vi "get_speed_params.vi"(8 "error in (no error)":errorcluster, 11 "TrajectoryDL090201FrameScan in":refnum<class "TrajectoryDL090201FrameScan.lvclass">) -> (0 "error out":errorcluster, 1 "line-scan time":dbl[unit]=-1.0, 2 "frame rate":dbl[unit]=-1.0, 3 "TrajectoryDL090201FrameScan out":refnum<class "TrajectoryDL090201FrameScan.lvclass">, 4 "pixel-dwell time":dbl[unit]=-1e-06)   [LabVIEW 2010, in "TrajectoryDL090201FrameScan.lvclass"]
uses:
  TrajectoryDL090201FrameScan.lvclass
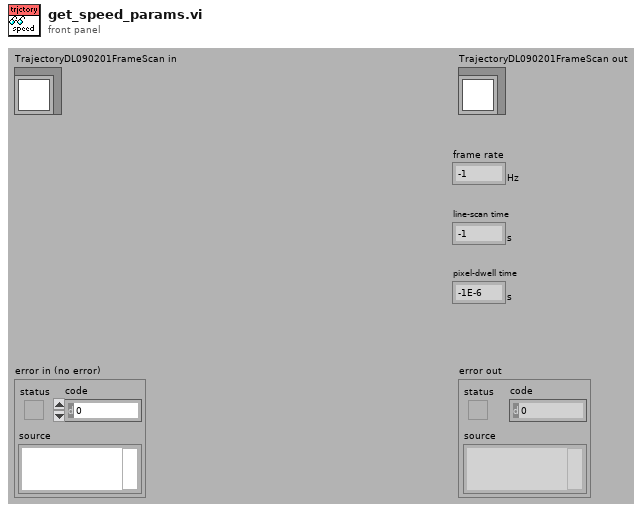
[diagram p1: front panel]
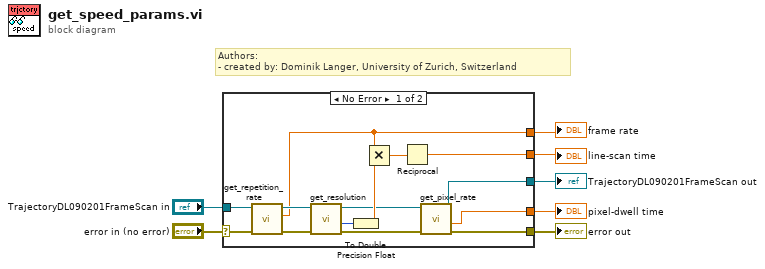
[diagram p0: block diagram]
diagram:
  # "Authors: \n- created by: Dominik Langer, University of Zurich, Switzerland"
  n1 = case shown="No Error" "error in (no error)" {
    selector: "error in (no error)" -> [w21 w23]
    tunnel: [w11 w23] -> w6
    tunnel: [w8 w22] -> w4
    tunnel: "TrajectoryDL090201FrameScan in" -> [w20 w22]
    tunnel: [w15 _] -> w3
    tunnel: [w13 _] -> w2
    tunnel: [w9 _] -> w1
    frame No Error {
      n2 = call-dynamic "get_repetition_rate.vi"("error in (no error)"=w21, "GenericTrajectory in"=w20) -> ("error out"=w18:errorcluster, "repetition rate"=w15:dbl[unit], "GenericTrajectory out"=w19:refnum<class "TrajectoryDL090201FrameScan.lvclass">)  [unwired: 7 in]
      n3 = call-dynamic "get_resolution.vi"("error in (no error)"=w18, "TrajectoryDL090201FrameScan in"=w19) -> ("error out"=w12:errorcluster, "y"=w17:i32, "TrajectoryDL090201FrameScan out"=w10:refnum<class "TrajectoryDL090201FrameScan.lvclass">)  [unwired: 6 in, 1 out]
      n4 = To Double Precision Float(number=w17) -> (double precision float=w16:dbl)
      n5 = Multiply(x=w15, y=w16) -> (x*y=w14:dbl[unit])
      n6 = Reciprocal(x=w14) -> (1/x=w13:dbl[unit])
      n7 = call-dynamic "get_pixel_rate.vi"("error in (no error)"=w12, "GenericTrajectory in"=w10) -> ("error out"=w11:errorcluster, "pixel dwell time"=w9:dbl[unit], "GenericTrajectory out"=w8:refnum<class "TrajectoryDL090201FrameScan.lvclass">)  [unwired: 6 in, 1 out]
    }
    frame Error {
    }
  }
  "error out" <- w6
  "TrajectoryDL090201FrameScan out" <- w4
  "frame rate" <- w3
  "line-scan time" <- w2
  "pixel-dwell time" <- w1
